vi "TrajetoryCreationAbsoluteSwerve.vi"(8 "End Pose  ENG":T1={"TRANSLATION"={"X"=0.0, "Y"=0.0}, "ROTATION"={"VALUE"=0.0, "COS"=1.0, "SIN"=0.0}} {"ROTATION"."SIN" format="%13.4f"; "ROTATION"."COS" format="%13.4f"; "ROTATION"."VALUE" format="%13.4f"; "TRANSLATION"."Y" format="%14.3f"; "TRANSLATION"."X" format="%14.3f"}, 9 "Current Pose SI":T1={"TRANSLATION"={"X"=0.0, "Y"=0.0}, "ROTATION"={"VALUE"=0.0, "COS"=1.0, "SIN"=0.0}} {"ROTATION"."SIN" format="%13.4f"; "ROTATION"."COS" format="%13.4f"; "ROTATION"."VALUE" format="%13.4f"; "TRANSLATION"."Y" format="%14.3f"; "TRANSLATION"."X" format="%14.3f"}, 10 "Max Velocity Ft/Sec":dbl=13.0 format="%17.3f", 11 "SWERVE_DRIVE_KINEMATICS":T4 {"SavedModuleStates"."Angle"."SIN" format="%13.4f"; "SavedModuleStates"."Angle"."COS" format="%13.4f"; "SavedModuleStates"."Angle"."VALUE" format="%13.4f"; "PrevCoR"."Y" format="%14.3f"; "PrevCoR"."X" format="%14.3f"; "Modules"."Y" format="%14.3f"; "Modules"."X" format="%14.3f"}) -> (0 "Trajectory  creation error":errorcluster, 1 "Absolute Trajectory":T7 {"States"."POSE"."ROTATION"."SIN" format="%13.4f"; "States"."POSE"."ROTATION"."COS" format="%13.4f"; "States"."POSE"."ROTATION"."VALUE" format="%13.4f"; "States"."POSE"."TRANSLATION"."Y" format="%14.3f"; "States"."POSE"."TRANSLATION"."X" format="%14.3f"; "TotalTImeSecs" format="%20.3f"}, 3 "TotalTImeSecs":dbl)   [LabVIEW 2023]
uses:
  <vilib>/Rock Robotics/WPI/ThirdParty/JAS_Junk/TrajLib/Enum/TRAJECTORY_SPLINE_TYPE_ENUM.ctl
  <vilib>/Rock Robotics/WPI/ThirdParty/JAS_Junk/TrajLib/TypeDef/TRAJECTORY.ctl
  <vilib>/Rock Robotics/WPI/ThirdParty/JAS_Junk/TrajLib/TypeDef/TRAJ_STATE.ctl
  <vilib>/Rock Robotics/WPI/ThirdParty/JAS_Junk/TrajLib/TypeDef/POSE2D.ctl
  <vilib>/Rock Robotics/WPI/ThirdParty/JAS_Junk/TrajLib/TypeDef/TRANSLATION2D.ctl
  <vilib>/Rock Robotics/WPI/ThirdParty/JAS_Junk/TrajLib/TypeDef/ROTATION2D.ctl
  <vilib>/Rock Robotics/WPI/ThirdParty/JAS_Junk/TrajLib/TypeDef/SWERVE_DRIVE_KINEMATICS.ctl
  <vilib>/Analysis/Matrix/Datatypes/RealMatrix.ctl
  <vilib>/Rock Robotics/WPI/ThirdParty/JAS_Junk/TrajLib/TypeDef/SWERVE_DRIVE_MODULE_STATE.ctl
  <vilib>/Rock Robotics/WPI/ThirdParty/JAS_Junk/TrajLib/SwerveDriveKinematicsConstraint_New.vi
  <vilib>/Rock Robotics/WPI/ThirdParty/JAS_Junk/TrajLib/TrajectoryConfig_AddConstraint.vi
  <vilib>/Rock Robotics/WPI/ThirdParty/JAS_Junk/TrajLib/CentripetalAccelConstraint_New.vi
  <vilib>/Rock Robotics/WPI/ThirdParty/JAS_Junk/TrajLib/Rotation2d_CreateAngle.vi
  <vilib>/Rock Robotics/WPI/ThirdParty/JAS_Junk/TrajLib/Translation2d_GetXY.vi
  <vilib>/Rock Robotics/WPI/ThirdParty/JAS_Junk/TrajLib/Rotation2d_CreateXY.vi
  <vilib>/Rock Robotics/WPI/ThirdParty/JAS_Junk/TrajLib/Util_CalcDist.vi
  <vilib>/Rock Robotics/WPI/ThirdParty/JAS_Junk/TrajLib/Trajectory_Library.lvlib
  <vilib>/Analysis/Matrix/NI_Matrix.lvlib
panel:
  in  "Spline Type":T9
  in  "Use Swerve Drive\nKinematic\nConstraint":bool=TRUE
  in  "Use Centripetal\nAcceleration\nConstaint":bool=TRUE
  out "MaxAcceleration  M/S^2":dbl=1.3 format="%17.4f"
  out "MaxVelocity M/S":dbl=2.0 format="%17.4f"
  out "Max Cent Accel":dbl=1.0 format="%20.4f"
  in  "Max Cent Accel INCHES/SEC^2":dbl=36.0 format="%20.1f"
  in  "MaxAcceleration INCHES/SEC^2":dbl=50.0 format="%17.1f"
  in  "MaxVelocity Fraction":dbl=0.8 format="%17.3f"
  # "This VI is designed to be called by BEGIN.VI, but can be executed directly to test trajectory parameters."
  # "CREATED TRAJECTORY INFORMATION"
  # "TRAJECTORY CONFIGURATION"
  # "real sim robot 20.9 inch"
  # "TRAJECTORY DEFINITION"
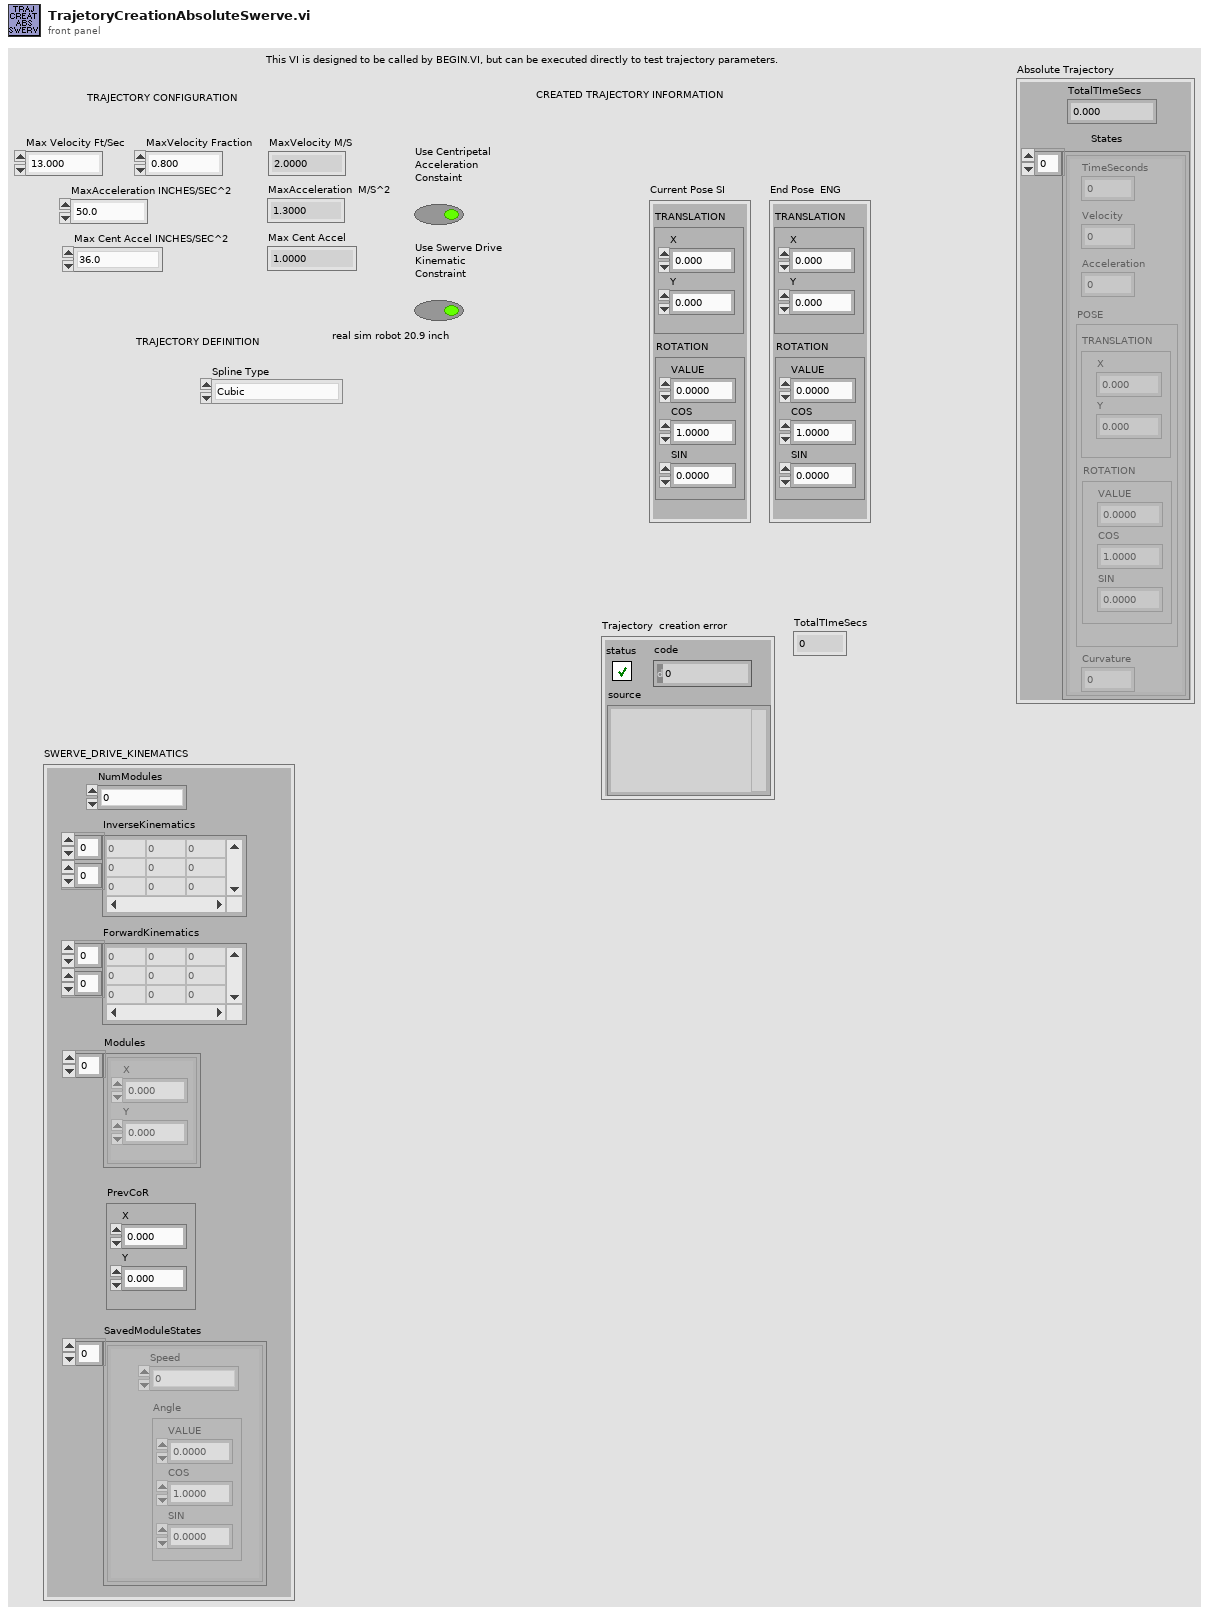
[diagram p1: front panel]
types:
  T1 = typedef "Trajectory_Library.lvlib/POSE2D.ctl" = cluster{"TRANSLATION":T2, "ROTATION":T3}
  T2 = typedef "Trajectory_Library.lvlib/TRANSLATION2D.ctl" = cluster{"X":dbl, "Y":dbl}
  T3 = typedef "Trajectory_Library.lvlib/ROTATION2D.ctl" = cluster{"VALUE":dbl, "COS":dbl, "SIN":dbl}
  T4 = typedef "Trajectory_Library.lvlib/SWERVE_DRIVE_KINEMATICS.ctl" = cluster{"NumModules":i32, "InverseKinematics":T5, "ForwardKinematics":T5, "Modules":T2[], "PrevCoR":T2, "SavedModuleStates":T6[]}
  T5 = typedef "NI_Matrix.lvlib/RealMatrix.ctl" = dbl[][]
  T6 = typedef "Trajectory_Library.lvlib/SWERVE_DRIVE_MODULE_STATE.ctl" = cluster{"Speed":dbl, "Angle":T3}
  T7 = typedef "Trajectory_Library.lvlib/TRAJECTORY.ctl" = cluster{"TotalTImeSecs":dbl, "States":T8[]}
  T8 = typedef "Trajectory_Library.lvlib/TRAJ_STATE.ctl" = cluster{"TimeSeconds":dbl, "Velocity":dbl, "Acceleration":dbl, "POSE":T1, "Curvature":dbl}
  T9 = typedef "Trajectory_Library.lvlib/TRAJECTORY_SPLINE_TYPE_ENUM.ctl" = enum16{"Cubic", "Cubic With Weights", "Quintic", "Quintic With Weights"}
  T10 = typedef "Trajectory_Library.lvlib/WEIGHTED_WAYPOINT.ctl" = cluster{"TRANSLATION":T2, "ROTATION":T3, "SCALAR":dbl}
  T11 = typedef "Trajectory_Library.lvlib/TRAJ_CONFIG.ctl" = cluster{"MaxVelocity":dbl, "Max Acceleration":dbl, "StartVelocity":dbl, "End Velocity":dbl, "Reversed":bool, "Constraints":variant[]}
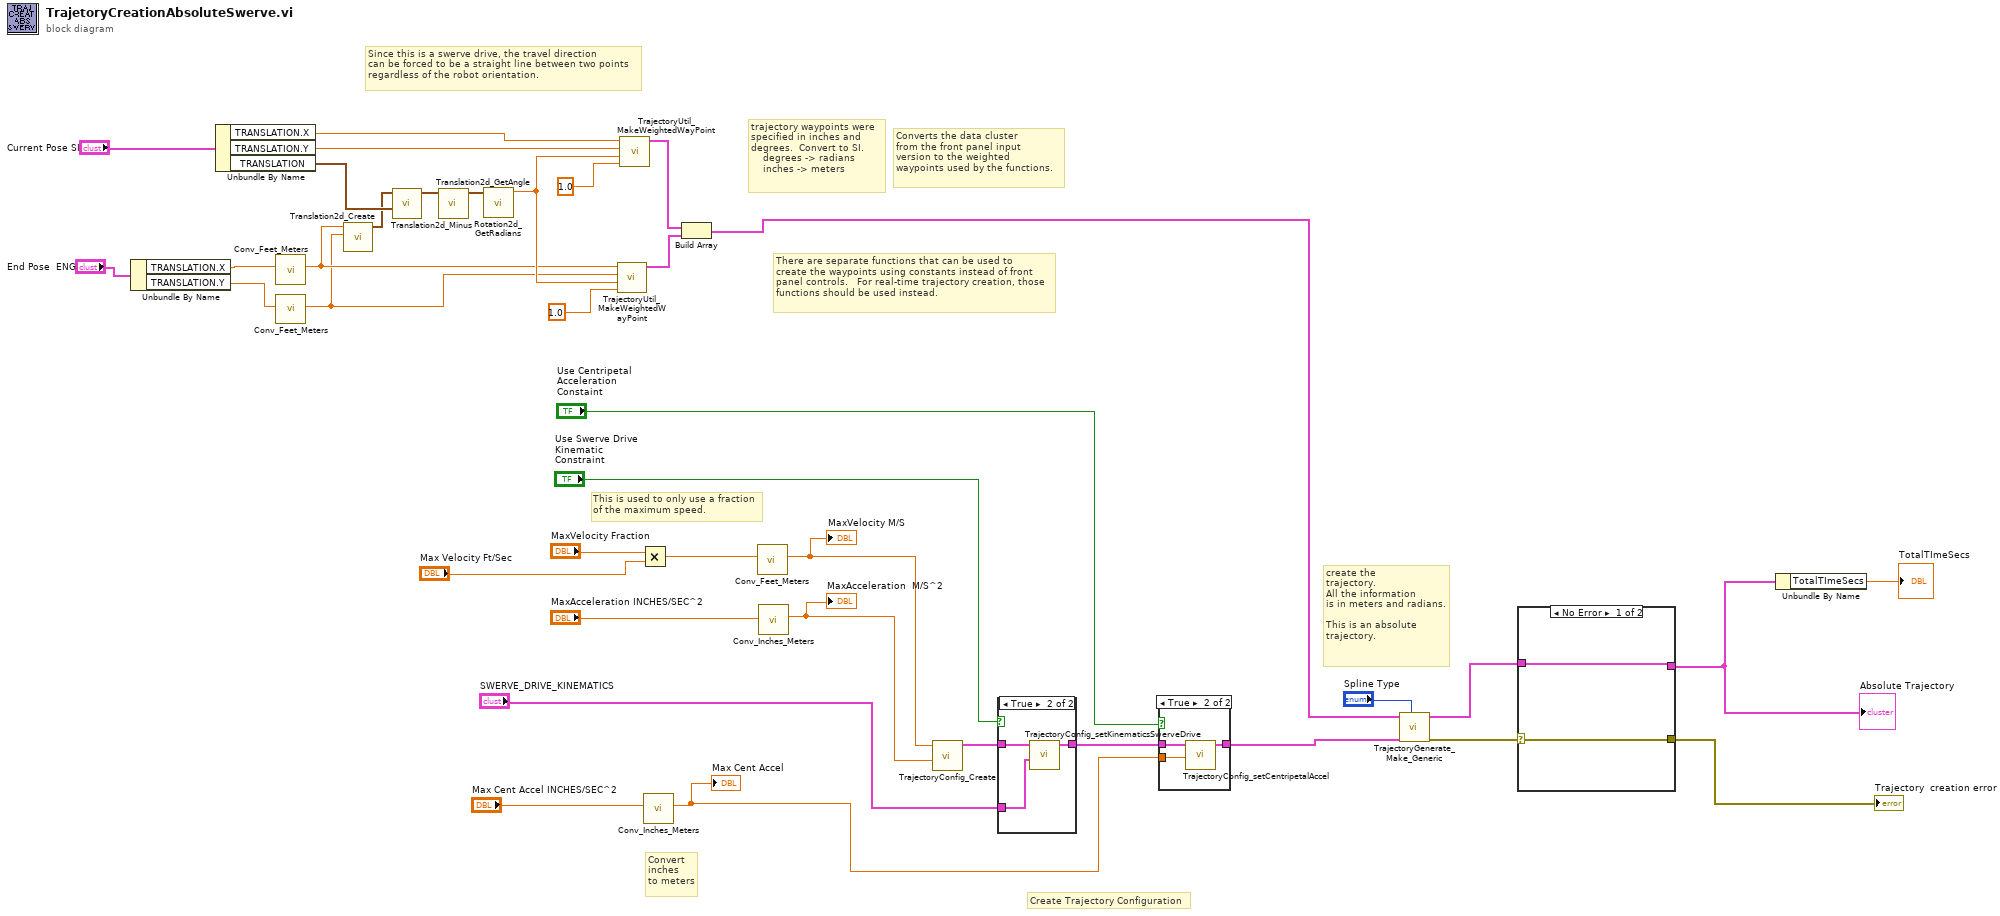
[diagram p0: block diagram]
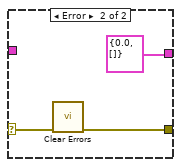
[diagram p2: hidden frame]
diagram:
  # "Since this is a swerve drive, the travel direction\ncan be forced to be a straight line between two points\nregardless of the robot orientation."
  # "There are separate functions that can be used to \ncreate the waypoints using constants instead of front\npanel controls.   For real-time trajectory creation, those\nfunctions should be used instead."
  # "This is used to only use a fraction\nof the maximum speed."
  # "Converts the data cluster\nfrom the front panel input\nversion to the weighted \nwaypoints used by the functions."
  # "Convert\ninches\nto meters"
  # "create the\ntrajectory.\nAll the information\nis in meters and radians.\n\nThis is an absolute \ntrajectory."
  # "trajectory waypoints were \nspecified in inches and\ndegrees.  Convert to SI.\n    degrees -> radians\n    inches -> meters"
  # "Create Trajectory Configuration"
  n1 = Unbundle By Name("End Pose  ENG") -> ("TRANSLATION.X"=w14:dbl, "TRANSLATION.Y"=w13:dbl)
  n2 = Unbundle By Name("Current Pose SI") -> ("TRANSLATION.X"=w20:dbl, "TRANSLATION.Y"=w19:dbl, "TRANSLATION"=w11:T2)
  n3 = call <vilib>:"Conv_Feet_Meters.vi"("Feet"=w14) -> ("Meters"=w7:dbl)  [unwired: 10 in]
  n4 = call <vilib>:"Conv_Feet_Meters.vi"("Feet"=w13) -> ("Meters"=w6:dbl)  [unwired: 10 in]
  n5 = call <vilib>:"Translation2d_Create.vi"("Y"=w6, "X"=w7) -> ("TRANSLATION"=w5:T2)  [unwired: 9 in]
  n6 = call <vilib>:"Translation2d_Minus.vi"("other Translation"=w11, "In Translation"=w5) -> ("Out Translation"=w10:T2)  [unwired: 9 in]
  n7 = call <vilib>:"Translation2d_GetAngle.vi"("In Translation"=w10) -> ("Angle_Rotation2d"=w9:T3)  [unwired: 10 in]
  n8 = call <vilib>:"Rotation2d_GetRadians.vi"("in ROTATION"=w9) -> ("AngleRadians"=w8:dbl)  [unwired: 10 in]
  n9 = call <vilib>:"TrajectoryUtil_MakeWeightedWayPoint.vi"("Weight"=1.0, "Travel Angle Radians"=w8, "Y_M"=w6, "X_M"=w7) -> ("WEIGHTED_WAYPOINT"=w16:T10)  [unwired: 7 in]
  n10 = call <vilib>:"TrajectoryUtil_MakeWeightedWayPoint.vi"("Weight"=1.0, "Travel Angle Radians"=w8, "Y_M"=w19, "X_M"=w20) -> ("WEIGHTED_WAYPOINT"=w21:T10)  [unwired: 7 in]
  n11 = Multiply(x="MaxVelocity Fraction", y="Max Velocity Ft/Sec") -> (x*y=w27:dbl)
  n12 = call <vilib>:"Conv_Inches_Meters.vi"("INCH"="Max Cent Accel INCHES/SEC^2") -> ("Meters"=w32:dbl)  [unwired: 10 in]
  "Max Cent Accel" <- w32
  n13 = Build Array(w21, w16) -> (w22:T10[])
  n14 = call <vilib>:"Conv_Feet_Meters.vi"("Feet"=w27) -> ("Meters"=w30:dbl)  [unwired: 10 in]
  "MaxVelocity M/S" <- w30
  n15 = call <vilib>:"Conv_Inches_Meters.vi"("INCH"="MaxAcceleration INCHES/SEC^2") -> ("Meters"=w31:dbl)  [unwired: 10 in]
  "MaxAcceleration  M/S^2" <- w31
  n16 = call <vilib>:"TrajectoryConfig_Create.vi"("MaxAcceleration"=w31, "MaxVelocity"=w30) -> ("TRAJECTORY_CONFIG"=w36:T11)  [unwired: 9 in]
  n17 = case shown="True" "Use Swerve Drive\nKinematic\nConstraint" {
    tunnel: w36 -> [w39 w42]
    tunnel: [w39 w41] -> w35
    tunnel: "SWERVE_DRIVE_KINEMATICS" -> [_ w40]
    frame False {
    }
    frame True {
      n18 = call <vilib>:"TrajectoryConfig_setKinematicsSwerveDrive.vi"("SWERVE_DRIVE_KINEMATICS"=w40, "inTRAJECTORY_CONFIG"=w42) -> ("outTRAJECTORY_CONFIG"=w41:T11)  [unwired: 9 in]
    }
  }
  n19 = case shown="True" "Use Centripetal\nAcceleration\nConstaint" {
    tunnel: w35 -> [w43 w46]
    tunnel: [w43 w45] -> w29
    tunnel: w32 -> [_ w44]
    frame False {
    }
    frame True {
      n20 = call <vilib>:"TrajectoryConfig_setCentripetalAccel.vi"("Max Cent Accel"=w44, "inTRAJECTORY_CONFIG"=w46) -> ("outTRAJECTORY_CONFIG"=w45:T11)  [unwired: 9 in]
    }
  }
  n21 = call <vilib>:"TrajectoryGenerate_Make_Generic.vi"("Spline Type"="Spline Type", "traj_config"=w29, "WeightedWayPoints"=w22) -> ("error out"=w4:errorcluster, "TRAJECTORY"=w3:T7)  [unwired: 7 in]
  n22 = case shown="No Error" w4 {
    selector: w4 -> [w47 w50]
    tunnel: w3 -> [w48 _]
    tunnel: [w48 T7 {"TotalTImeSecs"=0.0, "States"=[]} ("TRAJECTORY")] -> w2
    tunnel: [w47 w49] -> w1
    frame No Error {
    }
    frame Error {
      n23 = call <vilib>:"Clear Errors.vi"("error in (no error)"=w50) -> ("error out"=w49:errorcluster)  [unwired: 5 in, 1 out]
    }
  }
  "Trajectory  creation error" <- w1
  "Absolute Trajectory" <- w2
  n24 = Unbundle By Name(w2) -> ("TotalTImeSecs"=→"TotalTImeSecs":dbl)
